vi "Adder3.vi"() -> (8 "Adder3":refnum<class "Adder3.lvclass">)   [LabVIEW 2017, in "Adder3.lvclass"]
uses:
  Adder3.lvclass
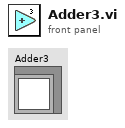
[diagram p1: front panel]
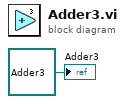
[diagram p0: block diagram]
diagram:
  "Adder3" <- refnum<class "Adder3.lvclass"> refnum ("Adder3.lvclass")
